vi "setActivePanel.vi"(8 "error in (no error)":errorcluster, 10 "Panel":refnum<class "Panel.lvclass">, 11 "UI in":refnum<class "UI.lvclass">) -> (0 "error out":errorcluster, 3 "UI out":refnum<class "UI.lvclass">)   [LabVIEW 2018, in "UI.lvclass"]
uses:
  UI.lvclass
  Panel/Panel.lvclass
  UI.lvclass/UI.ctl
  getPanel.vi
  setPanel.vi
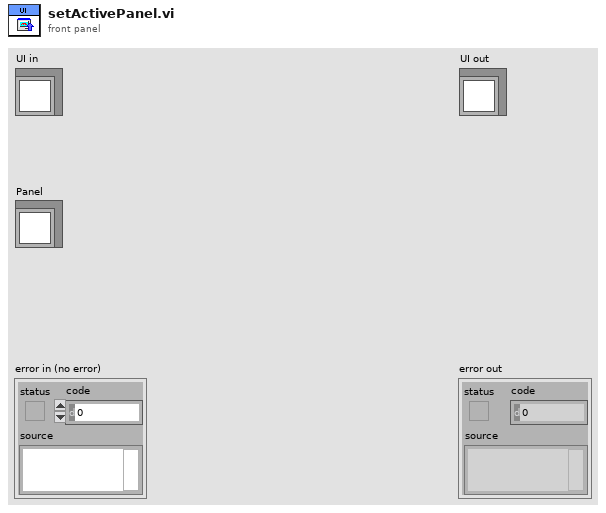
[diagram p1: front panel]
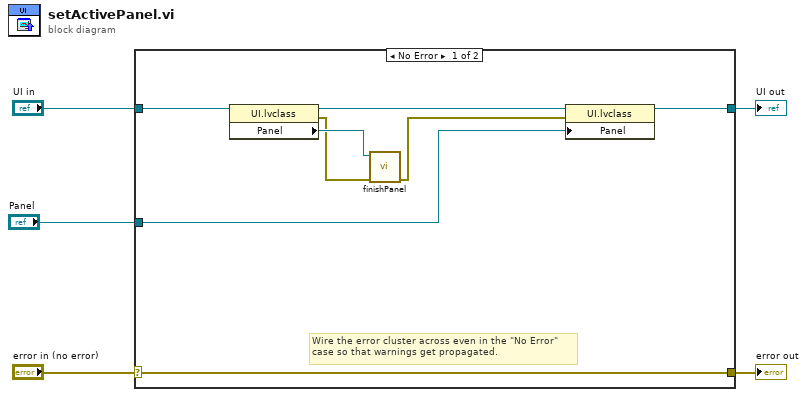
[diagram p0: block diagram]
diagram:
  n1 = case shown="No Error" "error in (no error)" {
    selector: "error in (no error)" -> [w12 w15]
    tunnel: [w12 w15] -> w4
    tunnel: [w11 w14] -> w2
    tunnel: "UI in" -> [w13 w14]
    tunnel: "Panel" -> [w8 _]
    frame No Error {
      # "Wire the error cluster across even in the \"No Error\"\ncase so that warnings get propagated."
      n2 = property class="UI.lvclass"(reference=w13) -> (reference out=w10:refnum<class "UI.lvclass">, error out=w6:errorcluster, "Panel"=w9:refnum<class "Panel.lvclass">)  [unwired: 1 in]
      n3 = call-dynamic "finishPanel.vi"("error in (no error)"=w6, "Panel in"=w9) -> ("error out"=w7:errorcluster)  [unwired: 9 in]
      n4 = property class="UI.lvclass"(reference=w10, error in=w7, "Panel"=w8) -> (reference out=w11:refnum<class "UI.lvclass">)  [unwired: 1 out]
    }
    frame Error {
    }
  }
  "error out" <- w4
  "UI out" <- w2
